vi "PH_Sound.evt PlayTone .vi"(0 "i ref in":refnum<vi>, 1 "Instance":string="N/A", 2 "Tone":T1 items=["c"=130.8, "cis"=138.6, "d"=146.8, "es"=155.6, "e"=164.8, "f"=174.6, "fis"=185.0, "g"=196.0, "as"=207.6, "a"=220.0, "b"=233.1, "h"=246.9, "c'"=261.6, "cis'"=277.2, "d'"=293.7, "es'"=311.1, "e'"=329.6, "f'"=349.2, "fis'"=370.0, "g'"=392.0, "as'"=415.3, "a'"=440.0, "b'"=466.2, "h'"=493.9, "c''"=523.3, "cis''"=554.4, "d''"=587.3, "es''"=622.3, "e''"=659.3, "f''"=689.5, "fis''"=740.0, "g''"=784.0, "as''"=830.6, "a''"=880.0, "b''"=932.3, "h''"=987.8, "c'''"=1047.0], 3 "Legth [ms]":i32, 5 "error in (no error)":errorcluster) -> (14 "i ref out":refnum<vi>, 19 "error out":errorcluster)   [LabVIEW 2014, in "PH_Sound.lvlib"]
doc: "This VI sends a command to play a tone"
uses:
  PH_Sound.lvlib
  PH_Sound.3Oktaves.ctl
  CS_Core/CSSystem/CoreLib/CoreLib.int 2 byte array.vi
  CS_Core/CSSystem/CoreLib/CoreLib.double 2 byte array.vi
  CS_Core/BaseProcess/BaseProcess.lvlib
  CS_Core/CSSystem/CoreLib/CoreLib.lvlib
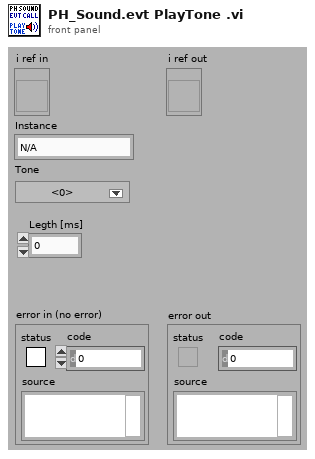
[diagram p1: front panel]
types:
  T1 = typedef "PH_Sound.lvlib/PH_Sound.3Oktaves.ctl" = dbl
  T2 = typedef "CoreDefs.rawDataType.ctl" = i8[]
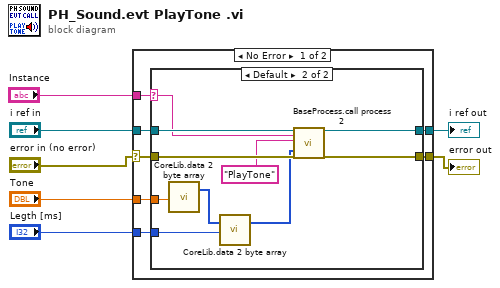
[diagram p0: block diagram]
diagram:
  n1 = case shown="No Error" "error in (no error)" {
    selector: "error in (no error)" -> [w9 w27]
    tunnel: [w14 w28] -> w7
    tunnel: [w13 w27] -> w6
    tunnel: "i ref in" -> [w12 w28]
    tunnel: "Instance" -> [w11 _]
    tunnel: "Tone" -> [w10 _]
    tunnel: "Legth [ms]" -> [w8 _]
    frame No Error {
      n2 = case shown="Default" w11 {
        selector: w11 -> [_ w22]
        tunnel: [w16 w26] -> w14
        tunnel: [w15 w25] -> w13
        tunnel: w12 -> [w16 w24]
        tunnel: w9 -> [w15 w23]
        tunnel: w10 -> [_ w21]
        tunnel: w8 -> [_ w19]
        frame "N/A" {
        }
        frame Default {
          n3 = call-poly "CoreLib.data 2 byte array.vi"("f64"=w21) -> ("byteArray out"=w18:T2)  [unwired: 18 in]
          n4 = call-poly "CoreLib.data 2 byte array.vi"("byteArray"=w18, "i32"=w19) -> ("byteArray out"=w17:T2)  [unwired: 17 in]
          n5 = call "BaseProcess.call process 2.vi"("i ref in"=w24, "Object"=w22, "Selector"="PlayTone", "Data"=w17, "error in (no error)"=w23) -> ("i ref out"=w26:refnum<vi>, "error out"=w25:errorcluster)  [unwired: 13 in]
        }
      }
    }
    frame Error {
    }
  }
  "error out" <- w6
  "i ref out" <- w7
